vi "Calibracion.vi"() -> ()   [LabVIEW 2015]
uses:
  <vilib>/Analysis/3filter.llb/Filter Passband Type.ctl
  <vilib>/Analysis/5stat.llb/RMS (DBL).vi
  <vilib>/Analysis/baseanly.llb/Mean (DBL).vi
  <vilib>/Analysis/3filter.llb/Butterworth Filter (DBL).vi
  <vilib>/measure/madcrms.llb/Basic Averaged DC-RMS for 1 Chan.vi
  <vilib>/measure/maspectr.llb/FFT Spectrum (Mag-Phase) for 1 Chan.vi
  <vilib>/measure/NI_MAPro.lvlib
  <vilib>/Analysis/NI_AALBase.lvlib
  <vilib>/Analysis/NI_AALPro.lvlib
panel:
  out "Waveform Graph":waveform(dbl)[](graph)
  out "Nuevo parámetro\nconfiguración":dbl
  out "RMS conseguido":dbl format="%0.2f"
  in  "Frecuencia de excitación\ndel patrón (Hz)":sgl=159.2
  in  "Aceleración del\npatrón (g RMS)":sgl=1.0
  out "% desviación\nfrecuencia":dbl
  in  "Carpeta donde están alojadas las señales del acelerómetro":path caption="file (use dialog)"
  in  "Nº del canal":i32
  out "DC de la señal":dbl format="%#_6e"
  out "Frecuencia de excitación\nVibrómetro  (Hz)":dbl
  out "Sensibilidad calibrada \n         (mV/g)":dbl
  in  "Parámetro de sensibilidad\n           (mV/g)":sgl=10.0
  in  "Frecuencia de muestreo":dbl=50000.0
  in  "Canales a calibrar (4 o 8)":u32=4
  # "INPUTS"
  # "OUTPUTS"
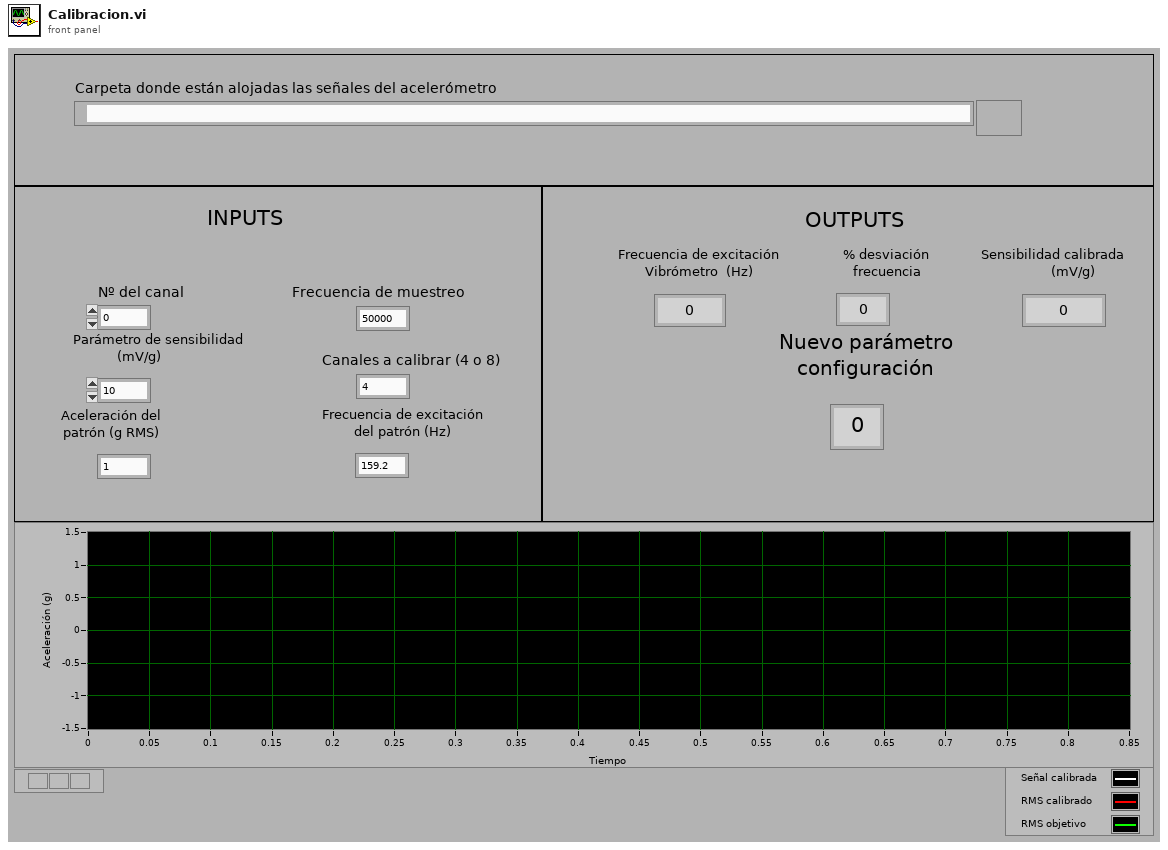
[diagram p1: front panel]
types:
  T1 = typedef "NI_AALBase.lvlib/Filter Passband Type.ctl" = enum32{"Lowpass", "Highpass", "Bandpass", "Bandstop"}
  T2 = enum16{"big-endian, network order", "native, host order", "little-endian"}
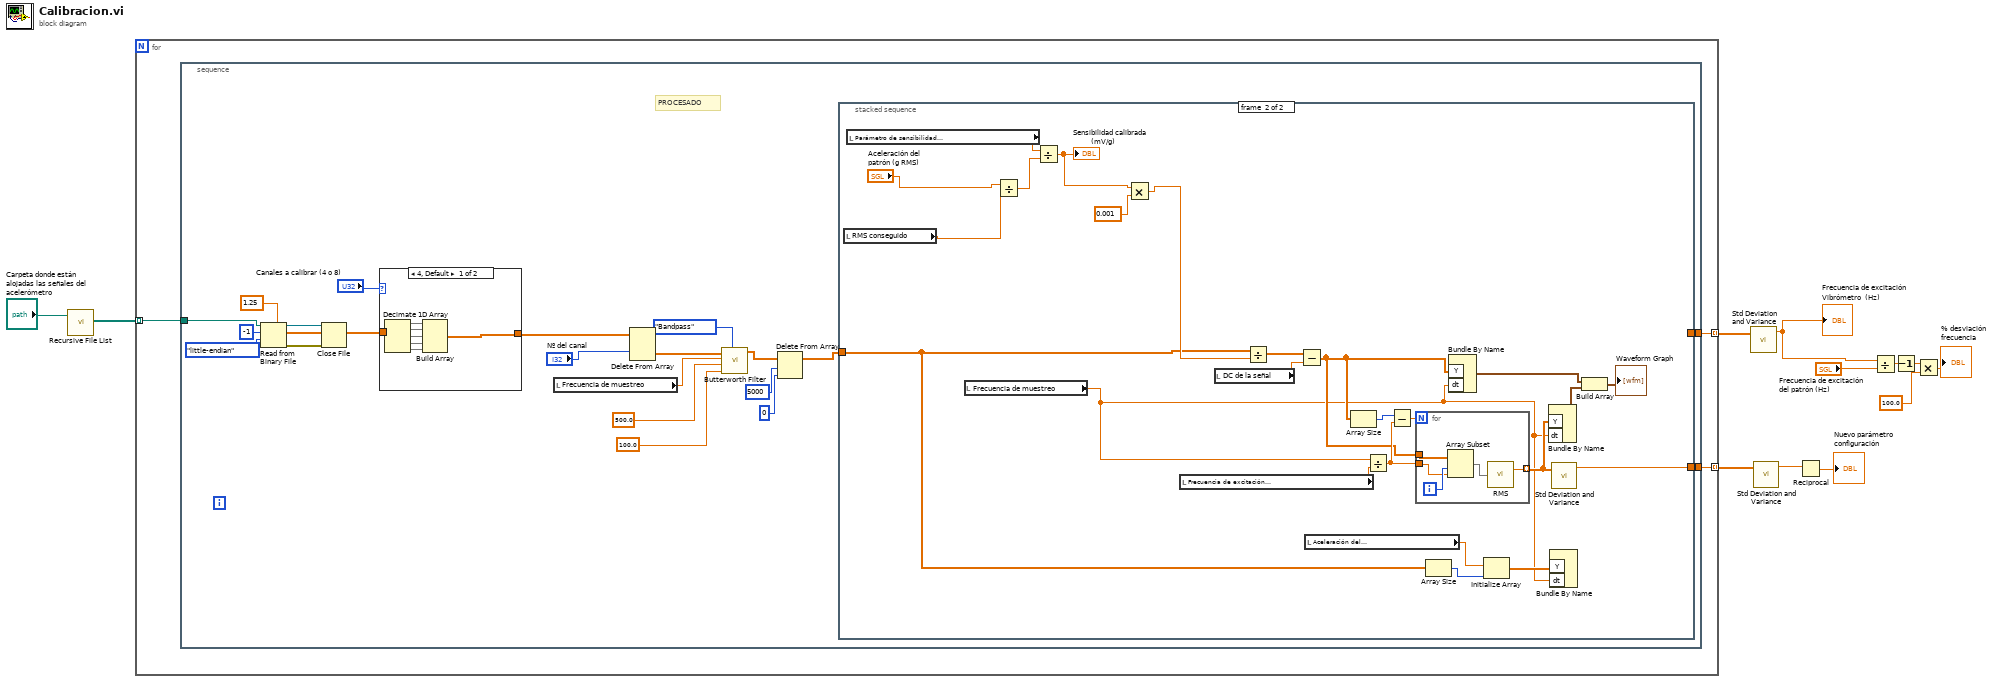
[diagram p0: block diagram]
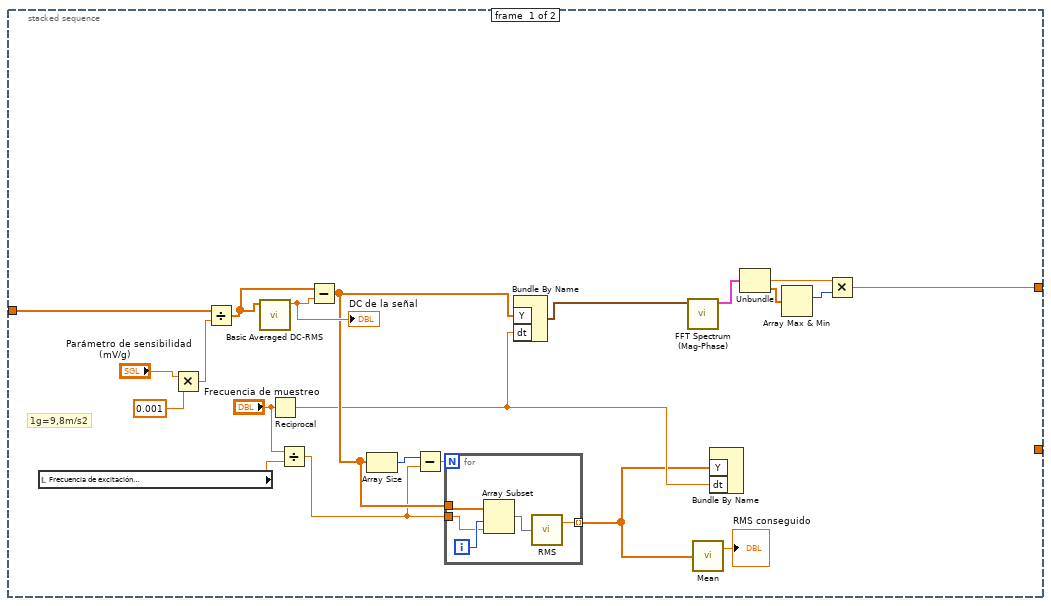
[diagram p2: hidden frame]
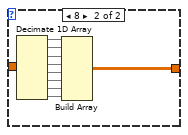
[diagram p3: hidden frame]
diagram:
  n1 = call <vilib>:"Recursive File List.vi"("Folder Path"="Carpeta donde están alojadas las señales del acelerómetro") -> ("All Files in Dir"=w11:path[])  [unwired: 6 in, 4 out]
  n2 = for {
    tunnel: [w15] -> w3 mode=indexing
    tunnel: w11 -> [w14] mode=indexing
    tunnel: [w13] -> w5 mode=indexing
    n3 = stacked-sequence {
      tunnel: [w18] -> w15
      tunnel: w14 -> [w17]
      tunnel: [w16] -> w13
      frame #0 {
        # "PROCESADO"
        n4 = Read from Binary File(5:sgl 1.25, 9:T2."little-endian" ("byte order (0:big-endian, network order)"), 10:-1 ("count (1)"), 11:w17) -> (0:w36:errorcluster, 2:w31:sgl[], 3:w33:refnum<file>)  [unwired: 1 in, 2 out]
        n5 = Close File(refnum=w33, error in=w36) -> ()  [unwired: 2 out]
        n6 = case shown="4, Default" "Canales a calibrar (4 o 8)" {
          tunnel: w31 -> [w95 w105]
          tunnel: [w94 w104] -> w30
          frame 4, Default {
            n7 = Decimate 1D Array(w95) -> (w97:sgl[], w98:sgl[], w96:sgl[], w93:sgl[], w92:sgl[])
            n8 = Build Array(w97, w98, w96, w93, w92) -> (w94:sgl[][])
          }
          frame 8 {
            n9 = Decimate 1D Array(w105) -> (w107:sgl[], w108:sgl[], w106:sgl[], w100:sgl[], w99:sgl[], w101:sgl[], w102:sgl[], w103:sgl[])
            n10 = Build Array(w107, w108, w106, w100, w99, w101, w102, w103) -> (w104:sgl[][])
          }
        }
        n11 = local read "Frecuencia de muestreo"() -> (w26:dbl)
        n12 = Delete From Array(array=w30, index (row)="Nº del canal") -> (deleted portion=w27:sgl[])  [unwired: 2 in, 1 out]
        n13 = call-poly <vilib>:"Butterworth Filter.vi"("filter type"=Filter_Passband_Type."Bandpass", "low cutoff freq: fl"=100.0, "high cutoff freq: fh"=500.0, "sampling freq: fs"=w26, "X"=w27) -> ("Filtered X"=w22:dbl[])  [unwired: 3 in, 1 out]
        n14 = Delete From Array(array=w22, length=5000, index=0) -> (array with subset deleted=w20:dbl[])  [unwired: 1 out]
        n15 = stacked-sequence {
          tunnel: w20 -> [w46 w63]
          tunnel: [_ w73] -> w18
          tunnel: [w37 _] -> w16
          frame #0 {
            # "1g=9,8m/s2"
            n16 = local read "Frecuencia de excitación\ndel patrón (Hz)"() -> (w42:sgl)
            n17 = Multiply(x="Parámetro de sensibilidad\n           (mV/g)", y=0.001) -> (x*y=w50:dbl)
            n18 = Divide(x=w46, y=w50) -> (x/y=w45:dbl[])
            n19 = call-poly <vilib>:"Basic Averaged DC-RMS.vi"("signal in"=w45) -> ("DC value"=w51:dbl)  [unwired: 7 in, 3 out]
            "DC de la señal" <- w51
            n20 = Reciprocal(x="Frecuencia de muestreo") -> (1/x=w40:dbl)
            n21 = Divide(x="Frecuencia de muestreo", y=w42) -> (x/y=w41:dbl)
            n22 = Subtract(x=w45, y=w51) -> (x-y=w44:dbl[])
            n23 = Array Size(array=w44) -> (size(s)=w47:i32)
            n24 = Subtract(x=w47, y=w41) -> (x-y=w48:dbl)
            n25 = for {
              N: w48 -> [_]
              tunnel: w41 -> [w59]
              tunnel: [w62] -> w39 mode=indexing
              tunnel: w44 -> [w61]
              i -> [w60]
              n26 = Array Subset(array=w61, index=w60, length=w59) -> (w58:dbl[])
              n27 = call-poly <vilib>:"RMS.vi"("X"=w58) -> ("rms value"=w62:dbl)  [unwired: 1 out]
            }
            n28 = Bundle By Name("Y"=w44, "dt"=w40) -> (w52:waveform(dbl))  [unwired: 1 in]
            n29 = call-poly <vilib>:"FFT Spectrum (Mag-Phase).vi"("time signal"=w52) -> ("magnitude"=w54:cluster{"f0":dbl, "df":dbl, "magnitude":dbl[]})  [unwired: 6 in, 4 out]
            n30 = call-poly <vilib>:"Mean.vi"("X"=w39) -> ("mean"=→"RMS conseguido":dbl)  [unwired: 1 out]
            n31 = Bundle By Name("Y"=w39, "dt"=w40) -> ()  [unwired: 1 in, 1 out]
            n32 = Unbundle(w54) -> ("df"=w55:dbl, "magnitude"=w56:dbl[])  [unwired: 1 out]
            n33 = Array Max & Min(array=w56) -> (max index (indices)=w57:i32)  [unwired: 3 out]
            n34 = Multiply(x=w55, y=w57) -> (x*y=w37:dbl)
          }
          frame #1 {
            n35 = local read "RMS conseguido"() -> (w82:dbl)
            n36 = local read "Parámetro de sensibilidad\n           (mV/g)"() -> (w85:sgl)
            n37 = local read "Frecuencia de muestreo"() -> (w65:dbl)
            n38 = Divide(x="Aceleración del\npatrón (g RMS)", y=w82) -> (x/y=w86:dbl)
            n39 = Divide(x=w85, y=w86) -> (x/y=w80:dbl)
            "Sensibilidad calibrada \n         (mV/g)" <- w80
            n40 = Multiply(x=w80, y=0.001) -> (x*y=w83:dbl)
            n41 = local read "Frecuencia de excitación\ndel patrón (Hz)"() -> (w75:sgl)
            n42 = local read "DC de la señal"() -> (w79:dbl)
            n43 = Divide(x=w63, y=w83) -> (x/y=w78:dbl[])
            n44 = Subtract(x=w78, y=w79) -> (x-y=w72:dbl[])
            n45 = local read "Aceleración del\npatrón (g RMS)"() -> (w64:sgl)
            n46 = Array Size(array=w72) -> (size(s)=w76:i32)
            n47 = Divide(x=w65, y=w75) -> (x/y=w74:dbl)
            n48 = Subtract(x=w76, y=w74) -> (x-y=w77:dbl)
            n49 = for {
              N: w77 -> [_]
              tunnel: w74 -> [w88]
              tunnel: [w91] -> w71 mode=indexing
              tunnel: w72 -> [w90]
              i -> [w89]
              n50 = Array Subset(array=w90, index=w89, length=w88) -> (w87:dbl[])
              n51 = call-poly <vilib>:"RMS.vi"("X"=w87) -> ("rms value"=w91:dbl)  [unwired: 1 out]
            }
            n52 = Array Size(array=w63) -> (size(s)=w67:i32)
            n53 = Bundle By Name("Y"=w72, "dt"=w65) -> (w68:waveform(dbl))  [unwired: 1 in]
            n54 = Initialize Array(w64, w67) -> (w66:sgl[])
            n55 = Bundle By Name("Y"=w71, "dt"=w65) -> (w69:waveform(dbl))  [unwired: 1 in]
            n56 = Bundle By Name("Y"=w66, "dt"=w65) -> ()  [unwired: 1 in, 1 out]
            n57 = call <vilib>:"Std Deviation and Variance.vi"("X"=w71) -> ("mean"=w73:dbl)  [unwired: 1 in, 2 out]
            n58 = Build Array(w68, w69) -> (→"Waveform Graph":waveform(dbl)[])
          }
        }
      }
    }
  }
  n59 = call <vilib>:"Std Deviation and Variance.vi"("X"=w5) -> ("mean"=w4:dbl)  [unwired: 1 in, 2 out]
  "Frecuencia de excitación\nVibrómetro  (Hz)" <- w4
  n60 = call <vilib>:"Std Deviation and Variance.vi"("X"=w3) -> ("mean"=w2:dbl)  [unwired: 1 in, 2 out]
  n61 = Reciprocal(x=w2) -> (1/x=→"Nuevo parámetro\nconfiguración":dbl)
  n62 = Divide(x=w4, y="Frecuencia de excitación\ndel patrón (Hz)") -> (x/y=w6:dbl)
  n63 = Decrement(x=w6) -> (x-1=w7:dbl)
  n64 = Multiply(x=w7, y=100.0) -> (x*y=→"% desviación\nfrecuencia":dbl)
